vi "Compare Dictionaries.vi"(8 "error in (no error)":errorcluster, 10 "Original Data (Dictionary)":T1[](array[typedef]), 11 "Converted Data (Dictionary)":T1[](array[typedef])) -> (0 "error out":errorcluster, 3 "Not Equal?":bool)   [LabVIEW 2016]
uses:
  Data/Typedefs/Dictionary--cluster.ctl
  <userlib>/_OpenG.lib/numeric/numeric.llb/Random Number Within Range - I32__ogtk.vi
  Data/Data.lvclass
panel:
  out "element":string
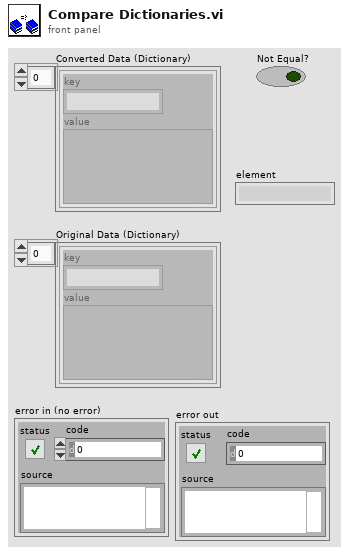
[diagram p1: front panel]
types:
  T1 = typedef "Data.lvclass/Dictionary--cluster.ctl" = cluster{"key":string, "value":variant}
  T2 = typedef "Dictionary Object RefNum__ogtk.ctl" = refnum<k1>
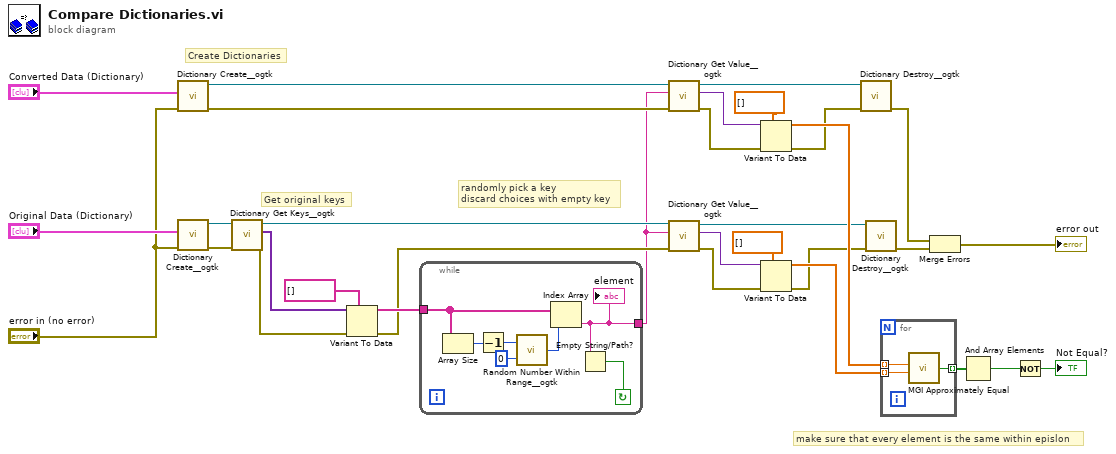
[diagram p0: block diagram]
diagram:
  # "make sure that every element is the same within epislon"
  # "randomly pick a key\ndiscard choices with empty key"
  # "Get original keys"
  # "Create Dictionaries"
  n1 = call <userlib>:"Dictionary Create__ogtk.vi"("error in (no error)"="error in (no error)", "initial dictionary (empty)"="Converted Data (Dictionary)") -> ("error out"=w20:errorcluster, "dictionary out"=w21:T2)  [unwired: 8 in]
  n2 = call <userlib>:"Dictionary Create__ogtk.vi"("error in (no error)"="error in (no error)", "initial dictionary (empty)"="Original Data (Dictionary)") -> ("error out"=w29:errorcluster, "dictionary out"=w30:T2)  [unwired: 8 in]
  n3 = call <userlib>:"Dictionary Get Keys__ogtk.vi"("error in (no error)"=w29, "dictionary"=w30) -> ("error out"=w26:errorcluster, "keys"=w25:variant[], "dictionary out"=w31:T2)  [unwired: 7 in]
  n4 = Variant To Data(error in=w26, type=string[] [], Variant=w25) -> (data=w32:string[], error out=w23:errorcluster)
  n5 = while {
    tunnel: w32 -> [w39]
    tunnel: [w33] -> w19
    stop <- w34 continue-if-true
    n6 = Array Size(array=w39) -> (size(s)=w36:i32)
    n7 = Decrement(x=w36) -> (x-1=w35:i32)
    n8 = call-poly <userlib>:"Random Number Within Range__ogtk.vi"("High"=w35, "Low"=0) -> ("Random Number"=w38:i32)  [unwired: 3 in]
    n9 = Index Array(array=w39, index=w38) -> (element=w33:string)
    "element" <- w33
    n10 = Empty String/Path?(string/path=w33) -> (empty?=w34:bool)
  }
  n11 = call <userlib>:"Dictionary Get Value__ogtk.vi"("error in"=w20, "key"=w19, "dictionary"=w21) -> ("error out"=w8:errorcluster, "value"=w18:variant, "dictionary out"=w9:T2)  [unwired: 5 in, 1 out]
  n12 = call <userlib>:"Dictionary Get Value__ogtk.vi"("error in"=w23, "key"=w19, "dictionary"=w31) -> ("error out"=w7:errorcluster, "value"=w2:variant, "dictionary out"=w10:T2)  [unwired: 5 in, 1 out]
  n13 = Variant To Data(error in=w8, type=dbl[] [], Variant=w18) -> (data=w16:dbl[], error out=w11:errorcluster)
  n14 = Variant To Data(error in=w7, type=dbl[] [], Variant=w2) -> (data=w17:dbl[], error out=w12:errorcluster)
  n15 = call <userlib>:"Dictionary Destroy__ogtk.vi"("error in (no error)"=w11, "dictionary"=w9) -> ("error out"=w5:errorcluster)  [unwired: 9 in]
  n16 = call <userlib>:"Dictionary Destroy__ogtk.vi"("error in (no error)"=w12, "dictionary"=w10) -> ("error out"=w6:errorcluster)  [unwired: 9 in]
  n17 = for {
    tunnel: w17 -> [w42] mode=indexing
    tunnel: w16 -> [w41] mode=indexing
    tunnel: [w40] -> w15 mode=indexing
    n18 = call <userlib>:"MGI Approximately Equal.vi"("Numeric 2"=w42, "Numeric 1"=w41) -> ("approx = ?"=w40:bool)  [unwired: 2 in]
  }
  n19 = Merge Errors(w5, w6) -> (→"error out":errorcluster)
  n20 = And Array Elements(Boolean array=w15) -> (logical AND=w14:bool)
  n21 = Not(x=w14) -> (.not. x?=→"Not Equal?":bool)
